vi "myRIOXC Trim String.vi"(9 "Max Length":i16=338, 10 "Text Font":T1, 11 "Input Text":string) -> (3 "Output Text":string)   [LabVIEW 2021]
uses:
  <vilib>/Utility/miscctls.llb/LVFontTypeDef.ctl
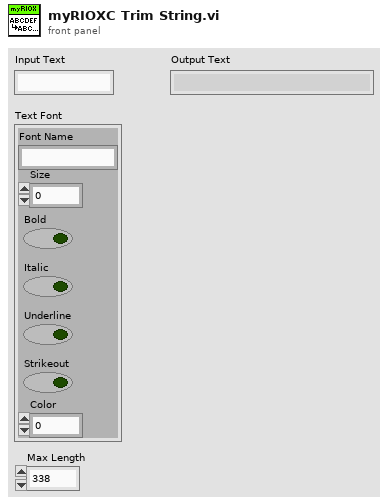
[diagram p1: front panel]
types:
  T1 = typedef "LVFontTypeDef.ctl" = cluster{"Font Name":string, "Size":u16, "Bold":bool, "Italic":bool, "Underline":bool, "Strikeout":bool, "Color":u32}
  T2 = cluster{"Font Name:":string, "Size":i16, "Strikeout?":bool, "Italic?":bool, "Underline?":bool, "Outline?":bool, "Shadow?":bool, "Bold?":bool}
  T3 = enum16{"User-specified Font", "Application Font", "System Font", "Dialog Font"}
  T4 = cluster{"left":i16, "top":i16, "right":i16, "bottom":i16}
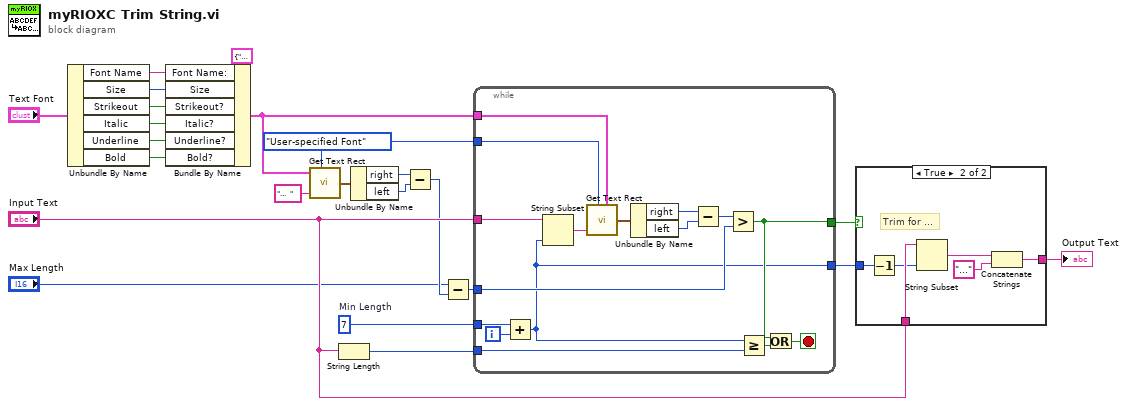
[diagram p0: block diagram]
diagram:
  w8 = T3."User-specified Font" ("desired font(Application)")
  w23 = 7  # Min Length
  n1 = Unbundle By Name("Text Font") -> ("Font Name"=w15:string, "Size"=w14:u16, "Strikeout"=w13:bool, "Italic"=w12:bool, "Underline"=w11:bool, "Bold"=w10:bool)
  n2 = Bundle By Name(cluster=T2 {"Font Name:"="", "Size"=0, "Strikeout?"=FALSE, "Italic?"=FALSE, "Underline?"=FALSE, "Outline?"=FALSE, "Shadow?"=FALSE, "Bold?"=FALSE} ("Font Info"), "Font Name:"=w15, "Size"=w14, "Strikeout?"=w13, "Italic?"=w12, "Underline?"=w11, "Bold?"=w10) -> (w7:T2)
  n3 = call <vilib>:"Get Text Rect.vi"("desired font(Application)"=w8, "text"="...  " ("string"), "[user-specified font]"=w7) -> ("rect"=w4:T4)  [unwired: 6 in]
  n4 = String Length(string="Input Text") -> (length=w22:i32)
  n5 = Unbundle By Name(w4) -> ("right"=w5:i16, "left"=w6:i16)
  n6 = Subtract(x=w5, y=w6) -> (x-y=w3:i16)
  n7 = Subtract(x="Max Length", y=w3) -> (x-y=w1:i16)
  n8 = while {
    tunnel: w7 -> [w36]
    tunnel: "Input Text" -> [w34]
    tunnel: w1 -> [w35]
    tunnel: w23 -> [w33]
    tunnel: w22 -> [w27]
    tunnel: [w29] -> w21
    tunnel: [w26] -> w20
    tunnel: w8 -> [w25]
    i -> [w32]
    stop <- w30 stop-if-true
    n9 = Add(x=w33, y=w32) -> (x+y=w26:i32)
    n10 = String Subset(string=w34, length (rest)=w26) -> (substring=w24:string)  [unwired: 1 in]
    n11 = call <vilib>:"Get Text Rect.vi"("desired font(Application)"=w25, "text"=w24, "[user-specified font]"=w36) -> ("rect"=w39:T4)  [unwired: 6 in]
    n12 = Unbundle By Name(w39) -> ("right"=w38:i16, "left"=w37:i16)
    n13 = Subtract(x=w38, y=w37) -> (x-y=w28:i16)
    n14 = Greater?(x=w28, y=w35) -> (0:w29:bool)
    n15 = Greater Or Equal?(x=w26, y=w27) -> (x >= y?=w31:bool)
    n16 = Or(x=w29, y=w31) -> (x .or. y?=w30:bool)
  }
  n17 = case shown="True" w21 {
    tunnel: w20 -> [_ w46]
    tunnel: "Input Text" -> [w40 w45]
    tunnel: [w40 w43] -> w18
    frame False {
      # "No need to trim"
    }
    frame True {
      # "Trim for ..."
      n18 = Decrement(x=w46) -> (x-1=w44:i32)
      n19 = String Subset(string=w45, length (rest)=w44) -> (substring=w42:string)  [unwired: 1 in]
      n20 = Concatenate Strings(w42, "..." ("string")) -> (w43:string)
    }
  }
  "Output Text" <- w18
